vi "Get_Saved_Pos_As_Number.vi"(0 "file path":path, 5 "file name":string="Motor_Positions_12.txt", 7 "Outuput Unit 1/2/3":T1=enum."Angle [TMC]", 9 "Outuput Unit 4":T1=enum."Angle [TMC]", 11 "error in":errorcluster, 13 "Microsteps (MS=64)":dbl=64.0) -> (4 "Pos 1":dbl, 6 "Pos 2":dbl, 8 "Pos 3":dbl, 10 "Pos 4":dbl, 15 "error out":errorcluster)   [LabVIEW 2018]
uses:
  ConversionAndInformation/Unit_Control.ctl
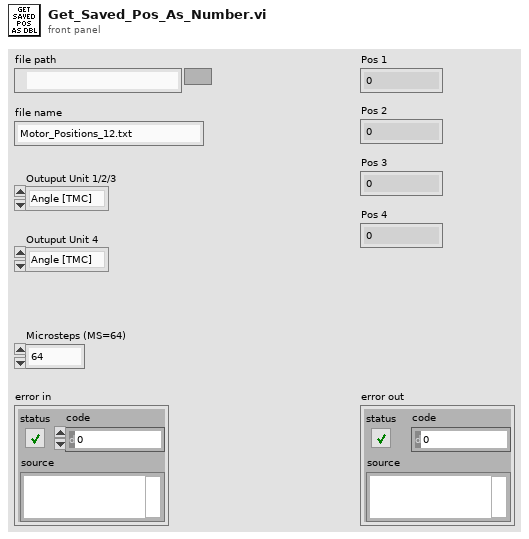
[diagram p1: front panel]
types:
  T1 = typedef "Unit_Control.ctl" = enum16{"Angle (Degrees)", "Rad", "Angle [TMC]", "Microsteps [TMC]", "Inches", "Nanometer", "Meter", "Centimeter", "Millimeter", "Micron"}
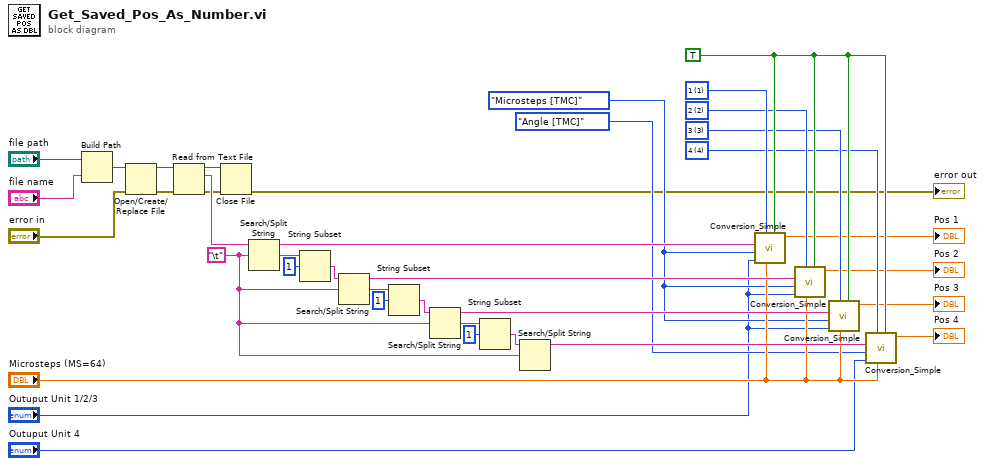
[diagram p0: block diagram]
diagram:
  w11 = Unit_Control."Microsteps [TMC]" ("Input Unit")
  w18 = u16 1 items=["none", "1", "2", "3", "4", "all"] ("Motor")
  w17 = u16 2 items=["none", "1", "2", "3", "4", "all"] ("Motor")
  w16 = u16 3 items=["none", "1", "2", "3", "4", "all"] ("Motor")
  w15 = u16 4 items=["none", "1", "2", "3", "4", "all"] ("Motor")
  w19 = TRUE ("Input = DBL/String (DBL[false])")
  w25 = "\t"
  n1 = Build Path(base path="file path", name or relative path="file name") -> (appended path=w38:path)
  n2 = Open/Create/Replace File(file path (use dialog)=w38, error in="error in") -> (refnum out=w36:refnum<file>, error out=w37:errorcluster)  [unwired: 4 in, 1 out]
  n3 = Read from Text File(file (use dialog)=w36, error in=w37) -> (refnum out=w3:refnum<file>, text=w24:string, error out=w2:errorcluster)  [unwired: 2 in, 1 out]
  n4 = Close File(refnum=w3, error in=w2) -> (error out=→"error out":errorcluster)  [unwired: 1 out]
  n5 = Search/Split String(string=w24, search string/char (-)=w25) -> (substring before match=w23:string, match + rest of string=w34:string)  [unwired: 1 in, 1 out]
  n6 = String Subset(string=w34, offset (0)=1) -> (substring=w33:string)  [unwired: 1 in]
  n7 = Search/Split String(string=w33, search string/char (-)=w25) -> (substring before match=w22:string, match + rest of string=w31:string)  [unwired: 1 in, 1 out]
  n8 = String Subset(string=w31, offset (0)=1) -> (substring=w30:string)  [unwired: 1 in]
  n9 = Search/Split String(string=w30, search string/char (-)=w25) -> (substring before match=w21:string, match + rest of string=w27:string)  [unwired: 1 in, 1 out]
  n10 = String Subset(string=w27, offset (0)=1) -> (substring=w26:string)  [unwired: 1 in]
  n11 = Search/Split String(string=w26, search string/char (-)=w25) -> (substring before match=w20:string)  [unwired: 1 in, 2 out]
  n12 = call "Conversion_Simple.vi"("Input = DBL/String (DBL[false])"=w19, "Microsteps (MS=64)"="Microsteps (MS=64)", "Motor"=w18, "Output Unit"="Outuput Unit 1/2/3", "Input Unit"=w11, "Input String"=w23) -> ("Output"=→"Pos 1":dbl)  [unwired: 4 in, 1 out]
  n13 = call "Conversion_Simple.vi"("Input = DBL/String (DBL[false])"=w19, "Microsteps (MS=64)"="Microsteps (MS=64)", "Motor"=w17, "Output Unit"="Outuput Unit 1/2/3", "Input Unit"=w11, "Input String"=w22) -> ("Output"=→"Pos 2":dbl)  [unwired: 4 in, 1 out]
  n14 = call "Conversion_Simple.vi"("Input = DBL/String (DBL[false])"=w19, "Microsteps (MS=64)"="Microsteps (MS=64)", "Motor"=w16, "Output Unit"="Outuput Unit 1/2/3", "Input Unit"=w11, "Input String"=w21) -> ("Output"=→"Pos 3":dbl)  [unwired: 4 in, 1 out]
  n15 = call "Conversion_Simple.vi"("Input = DBL/String (DBL[false])"=w19, "Microsteps (MS=64)"="Microsteps (MS=64)", "Motor"=w15, "Output Unit"="Outuput Unit 4", "Input Unit"=Unit_Control."Angle [TMC]", "Input String"=w20) -> ("Output"=→"Pos 4":dbl)  [unwired: 4 in, 1 out]
